vi "l_matr_v2.vi"() -> ()   [LabVIEW 2009]
panel:
  out "Linia selectata":bool[](array[boolean])=[FALSE, FALSE, TRUE, TRUE, FALSE]
  in  "Array 3":bool[][](array[boolean])=[[FALSE, TRUE, TRUE, TRUE, FALSE], [TRUE, FALSE, FALSE, FALSE, TRUE], [FALSE, FALSE, FALSE, FALSE, TRUE], [FALSE, FALSE, TRUE, TRUE, FALSE], [FALSE, FALSE, FALSE, FALSE, TRUE], [TRUE, FALSE, FALSE, FALSE, TRUE], [FALSE, TRUE, TRUE, TRUE, FALSE]]
  out "Linia":u8(slide)=3 scale=6.0..0.0
  in  "Iesire":bool
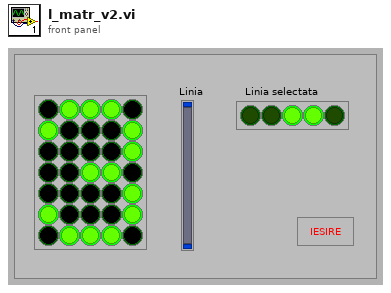
[diagram p1: front panel]
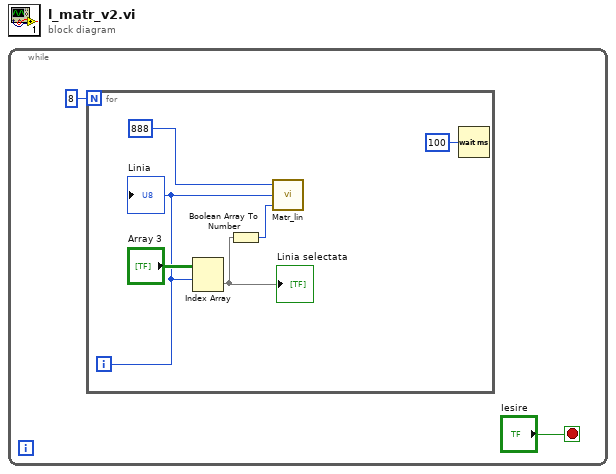
[diagram p0: block diagram]
diagram:
  n1 = while {
    stop <- "Iesire" stop-if-true
    n2 = for {
      N: 8 -> [_]
      i -> [w3]
      n3 = Index Array(array="Array 3", index (row)=w3) -> (element=w4:bool[])  [unwired: 1 in]
      "Linia selectata" <- w4
      n4 = Boolean Array To Number(Boolean array=w4) -> (number=w5:u32)
      n5 = call "Matr_lin.vi"("Date"=w5, "Linia"=w3, "Adresa port paralel"=888) -> ()  [unwired: 2 out]
      n6 = Wait (ms)(milliseconds to wait=u32 100) -> ()  [unwired: 1 out]
      "Linia" <- w3
    }
  }
